vi "tap_tri_wave.vi"() -> ()   [LabVIEW 2014]
panel:
  in  "Max Power (uW/mm^2)":dbl
  in  "Min Power (uW/mm^2)":dbl
  in  "period (frames)":dbl
  in  "Initial Power (uW/mm^2)":dbl
  in  "Hold Time (frames)":i32
  in  "period  (frames)":i32
  in  "Trials Per Voltage":i32
  in  "Array":dbl[](array[numeric])
  in  "Min Voltage":dbl
  out "Frames":i32
  in  "Transfer and Run Date Folder After Experiment":bool
  in  "SSH user name":string
  in  "SSH password":string
  in  "Wait before recording (s)":dbl
  in  "Tags":string
  in  "Start Recording":bool
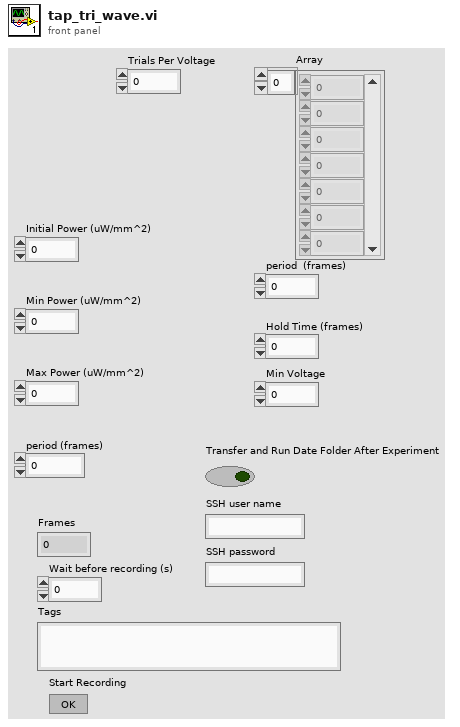
[diagram p1: front panel]
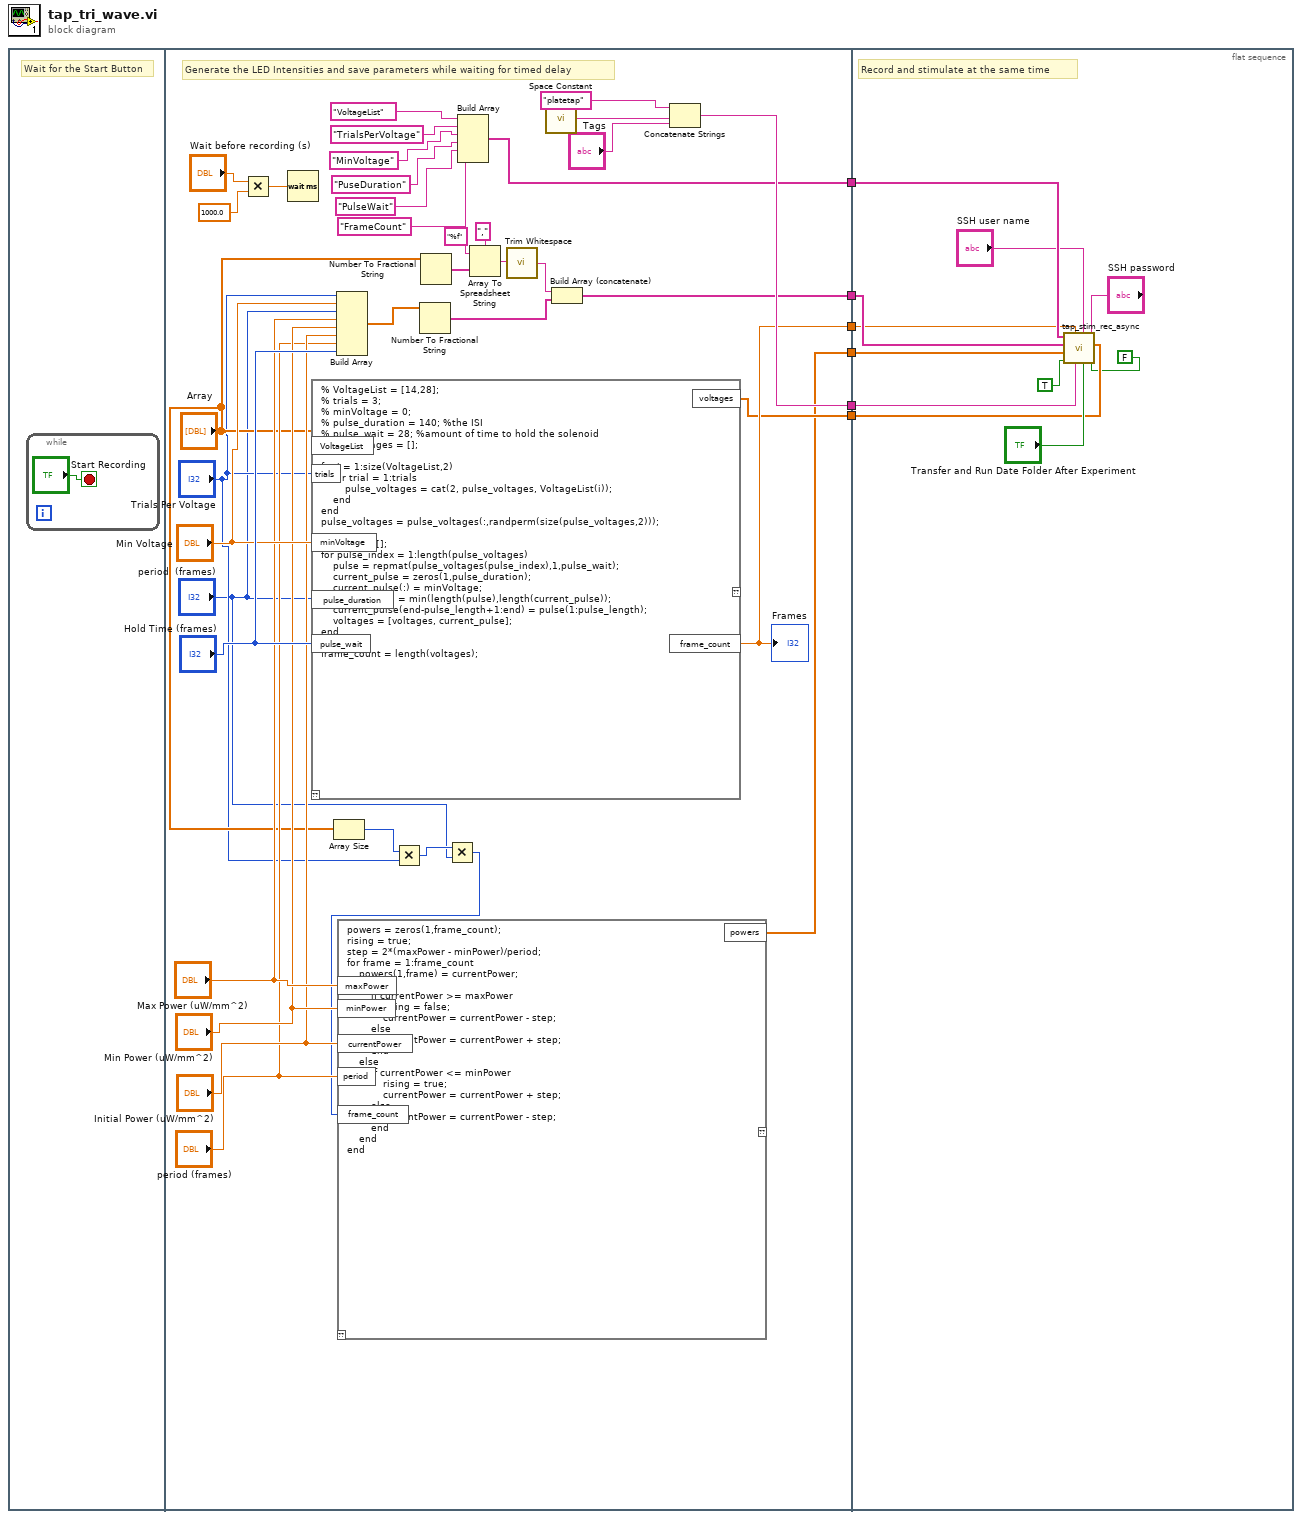
[diagram p0: block diagram]
diagram:
  n1 = flat-sequence {
    tunnel: [w41] -> w6
    tunnel: [w25] -> w5
    tunnel: [w35] -> w4
    tunnel: [w20] -> w3
    tunnel: [w9] -> w2
    tunnel: [w8] -> w1
    tunnel: w6 -> [w55]
    tunnel: w5 -> [w54]
    tunnel: w4 -> [w50]
    tunnel: w3 -> [w49]
    tunnel: w2 -> [w48]
    tunnel: w1 -> [w47]
    frame #0 {
      # "Wait for the Start Button"
      n2 = while {
        stop <- "Start Recording" stop-if-true
      }
    }
    frame #1 {
      # "Generate the LED Intensities and save parameters while waiting for timed delay"
      n3 = Multiply(x="Wait before recording (s)", y=1000.0) -> (x*y=w39:dbl)
      n4 = Wait (ms)(milliseconds to wait=w39) -> ()  [unwired: 1 out]
      n5 = script code="% VoltageList = [14,28];\n% trials = 3;\n% minVoltage = 0;\n% pulse_duration = 140; %the ISI\n% pulse_wait = 28; %amount of time to hold the solenoid\npulse_voltages = [];\n\nfor i = 1:size(VoltageList,2)\n    for trial = 1:trials\n        pulse_voltages = cat(2, pulse_voltages, VoltageList(i));\n    end\nend\npulse_voltages = pulse_voltages(:,randperm(size(pulse_voltages,2)));\n\nvoltages = [];\nfor pulse_index = 1:length(pulse_voltages)\n    pulse = repmat(pulse_voltages(pulse_index),1,pulse_wait);\n    current_pulse = zeros(1,pulse_duration);\n    current_pulse(:) = minVoltage;\n    pulse_length = min(length(pulse),length(current_pulse));\n    current_pulse(end-pulse_length+1:end) = pulse(1:pulse_length);\n    voltages = [voltages, current_pulse];\nend\n\nframe_count = length(voltages);"("pulse_duration"="period  (frames)", "trials"="Trials Per Voltage", "minVoltage"="Min Voltage", "VoltageList"="Array", "pulse_wait"="Hold Time (frames)") -> ("voltages"=w9:dbl[], "frame_count"=w20:dbl)  [unwired: 1 in, 1 out]
      "Frames" <- w20
      n6 = Array Size(array="Array") -> (size(s)=w14:i32)
      n7 = Build Array("Trials Per Voltage", "Min Voltage", "period  (frames)", "Max Power (uW/mm^2)", "Min Power (uW/mm^2)", "Initial Power (uW/mm^2)", "period (frames)", "Hold Time (frames)") -> (w24:dbl[])
      n8 = Multiply(x=w14, y="Trials Per Voltage") -> (x*y=w12:i32)
      n9 = Number To Fractional String(number=w24) -> (F-format string=w36:string[])  [unwired: 3 in]
      n10 = Number To Fractional String(number="Array") -> (F-format string=w23:string[])  [unwired: 3 in]
      n11 = Multiply(x=w12, y="period  (frames)") -> (x*y=w10:i32)
      n12 = script code="powers = zeros(1,frame_count);\nrising = true;\nstep = 2*(maxPower - minPower)/period;\nfor frame = 1:frame_count\n    powers(1,frame) = currentPower;\n    if rising\n        if currentPower >= maxPower\n            rising = false;\n            currentPower = currentPower - step;\n        else\n            currentPower = currentPower + step;\n        end\n    else\n        if currentPower <= minPower\n            rising = true;\n            currentPower = currentPower + step;\n        else\n            currentPower = currentPower - step;\n        end\n    end\nend"("currentPower"="Initial Power (uW/mm^2)", "frame_count"=w10, "period"="period (frames)", "minPower"="Min Power (uW/mm^2)", "maxPower"="Max Power (uW/mm^2)") -> ("powers"=w8:dbl[])  [unwired: 1 in, 1 out]
      n13 = Build Array("VoltageList", "TrialsPerVoltage", "MinVoltage", "PuseDuration", "PulseWait", "FrameCount") -> (w25:string[])
      n14 = Array To Spreadsheet String(delimiter (Tab)=",", array=w23, 3:"%f") -> (spreadsheet string=w33:string)
      n15 = call <vilib>:"Trim Whitespace.vi"("string"=w33) -> ("trimmed string"=w32:string)  [unwired: 1 in]
      n16 = call <vilib>:"Space Constant.vi"() -> ("String"=w43:string)
      n17 = Build Array (concatenate)(w32, w36) -> (w35:string[])
      n18 = Concatenate Strings("platetap", w43, "Tags") -> (w41:string)
    }
    frame #2 {
      # "Record and stimulate at the same time"
      n19 = call "tap_stim_rec_async.vi"("Convert Power to Voltage B"=FALSE, "voltages/power B"=w48, "SSH password"="SSH password", "Transfer and Run Date Folder After Experiment"="Transfer and Run Date Folder After Experiment", "SSH user name"="SSH user name", "Tags"=w55, "Frames"=w49, "Convert Power to Voltage"=TRUE, "voltages/power A"=w47, "parameters"=w50, "parameters headers"=w54) -> ()  [unwired: 1 in]
    }
  }
